vi "TDelay_bin.vi"(5 "Boolean":bool, 7 "delay":i32=1, 11 "error in":errorcluster) -> (6 "output":bool, 15 "error out":errorcluster)   [LabVIEW 2022 SP3]
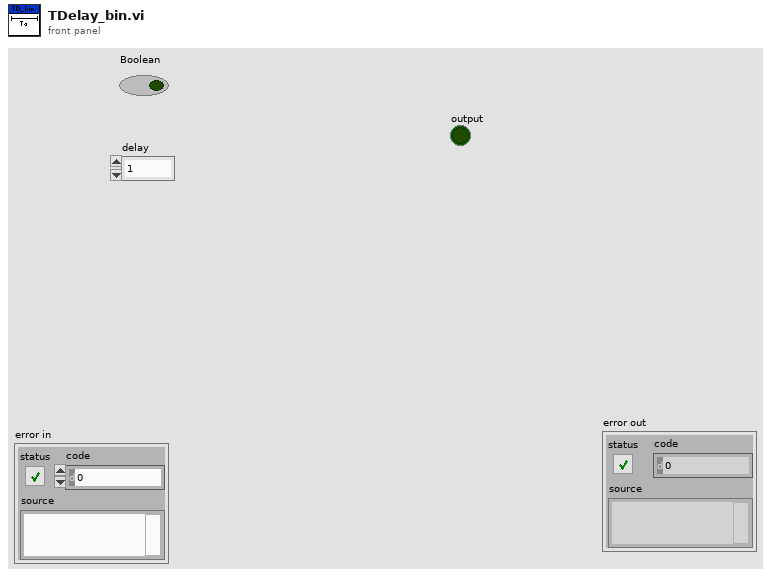
[diagram p1: front panel]
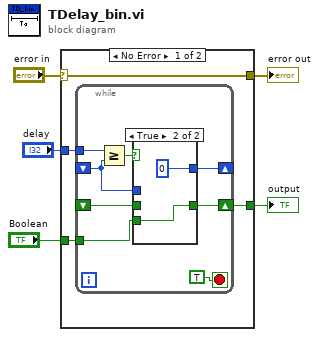
[diagram p0: block diagram]
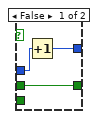
[diagram p2: hidden frame]
diagram:
  n1 = case shown="No Error" "error in" {
    selector: "error in" -> [w7 w23]
    tunnel: "Boolean" -> [w8 _]
    tunnel: "delay" -> [w9 _]
    tunnel: [w7 w23] -> w2
    tunnel: [w6 _] -> w1
    frame No Error {
      n2 = while {
        tunnel: w9 -> [w16]
        shift-right: [w14] -> _
        shift-left: _ -> [w15]
        shift-right: [w12] -> w6
        shift-left: _ -> [w10]
        tunnel: w8 -> [w11]
        stop <- TRUE stop-if-true
        n3 = Greater Or Equal?(x=w16, y=w15) -> (x >= y?=w13:bool)
        n4 = case shown="True" w13 {
          tunnel: w15 -> [w20 _]
          tunnel: [w19 0 ("delay")] -> w14
          tunnel: [w18 w21] -> w12
          tunnel: w11 -> [_ w21]
          tunnel: w10 -> [w18 _]
          frame False {
            n5 = Increment(x=w20) -> (x+1=w19:i32)
          }
          frame True {
          }
        }
      }
    }
    frame Error {
    }
  }
  "error out" <- w2
  "output" <- w1
